vi "VI server_Set Controls Property from String Format_Array Input.vi"(4 "Property":T1="Value", 7 "Labels":string[](array[string]), 8 "error in (no error)":errorcluster, 9 "Values":string[](array[string]), 11 "VI Server.RefsCluster":T2 caption="VI Server Cluster") -> (0 "error out":errorcluster, 3 "VI Server Cluster.DUP":T2)   [LabVIEW 2020]
doc: "Sets specified property of the multiple controls (labels array input) to values formatted as strings."
uses:
  VI Server_TypeDefs/VI Server_RefsCluster.ctl
  VI Server Libraries/VI Server Controls.llb/VI Server_Properties.ctl
  VI Server Toolkit LV2013.lvlib
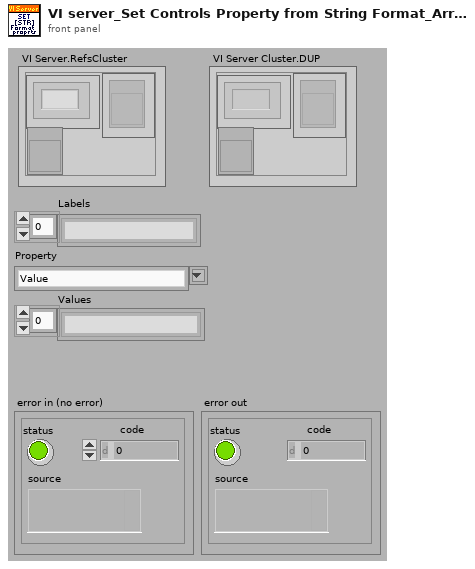
[diagram p1: front panel]
types:
  T1 = typedef "VI Server Toolkit LV2013.lvlib/VI Server_Properties.ctl" = string
  T2 = typedef "VI Server_RefsCluster.ctl" = cluster{"Labels":string[], "Refs":refnum<vi>[], "VI Ref":refnum<vi>}
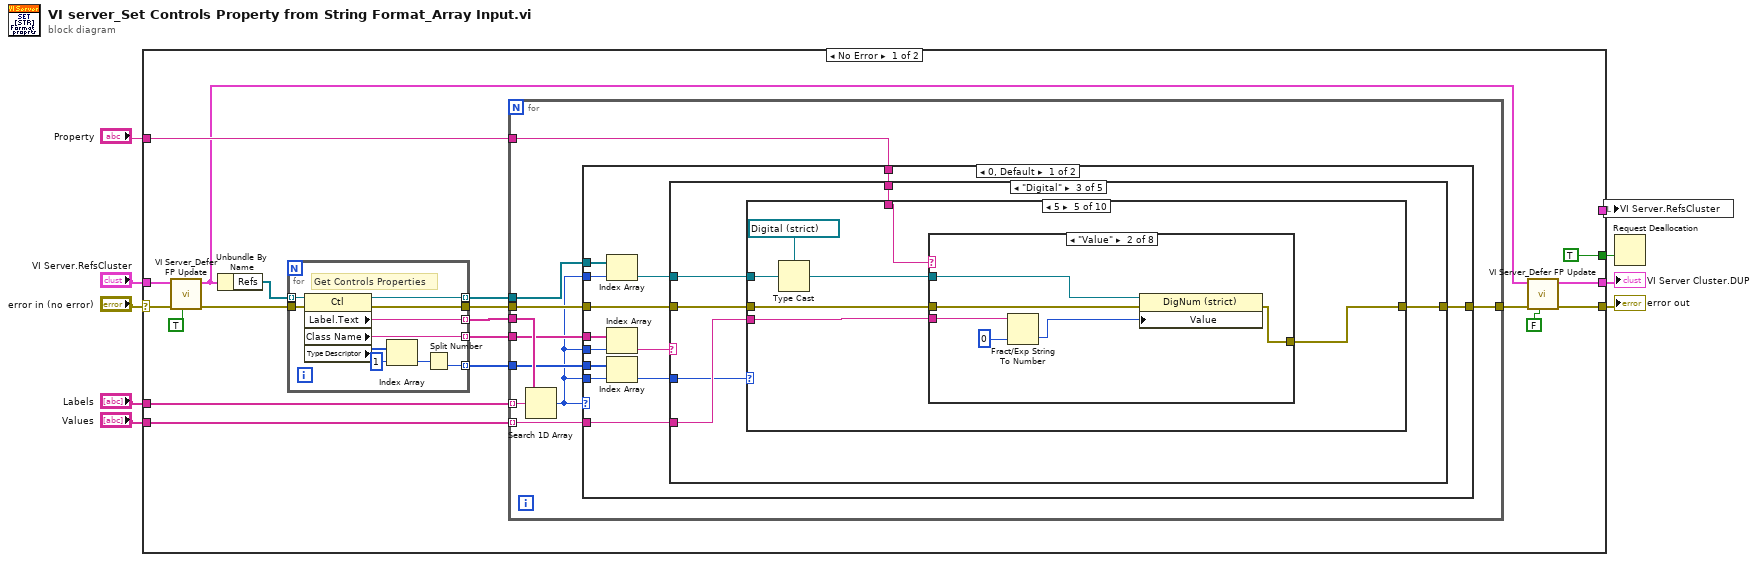
[diagram p0: block diagram]
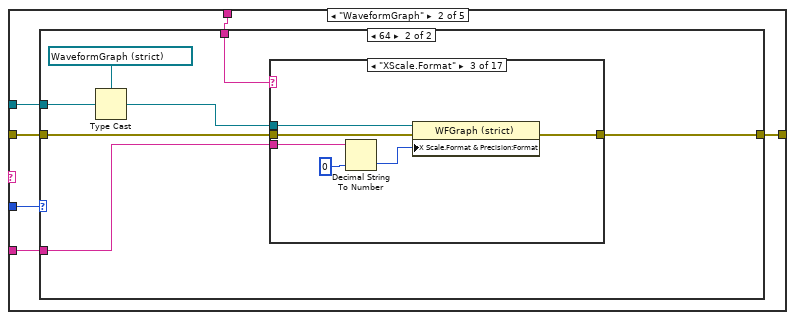
[diagram p3: hidden frame]
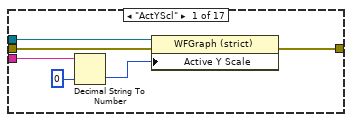
[diagram p5: hidden frame]
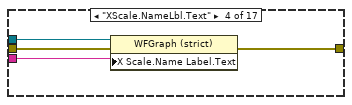
[diagram p7: hidden frame]
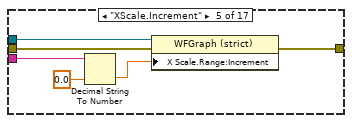
[diagram p8: hidden frame]
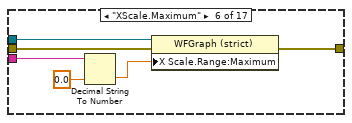
[diagram p9: hidden frame]
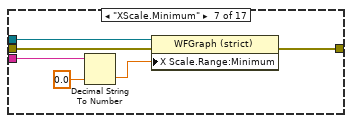
[diagram p10: hidden frame]
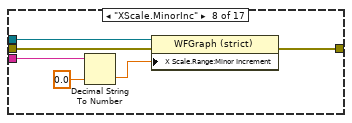
[diagram p11: hidden frame]
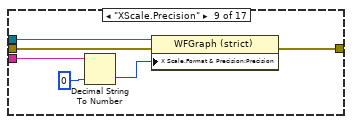
[diagram p12: hidden frame]
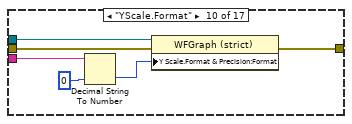
[diagram p13: hidden frame]
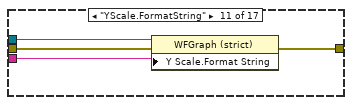
[diagram p14: hidden frame]
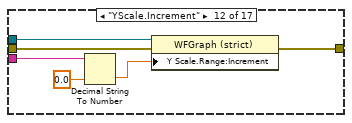
[diagram p15: hidden frame]
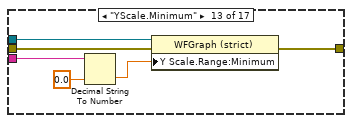
[diagram p16: hidden frame]
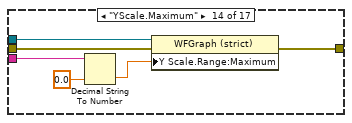
[diagram p17: hidden frame]
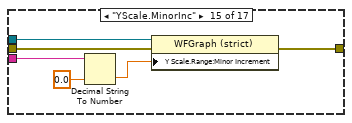
[diagram p18: hidden frame]
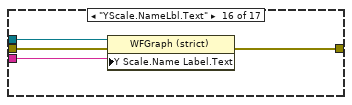
[diagram p19: hidden frame]
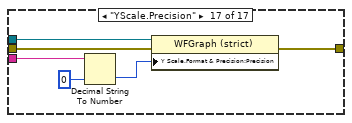
[diagram p20: hidden frame]
diagram:
  n1 = case shown="No Error" "error in (no error)" {
    selector: "error in (no error)" -> [w20 w1359]
    tunnel: "Labels" -> [w22 _]
    tunnel: "Values" -> [w23 _]
    tunnel: [w16 w1359] -> w7
    tunnel: "VI Server.RefsCluster" -> [w18 _]
    tunnel: "Property" -> [w13 _]
    tunnel: [w12 _] -> w3
    tunnel: [TRUE _] -> w2
    tunnel: [_ w1358] -> w1
    frame No Error {
      n2 = call "VI Server_Defer FP Update.vi"("Defer Panel Updates? (F)"=TRUE ("Defer Panel Updates (F)"), "error in"=w20, "VI Server Cluster"=w18) -> ("error out"=w19:errorcluster, "VI Server Cluster.DUP"=w10:T2)  [unwired: 7 out]
      n3 = Unbundle By Name(w10) -> ("Refs"=w21:refnum<vi>[])
      n4 = for {
        tunnel: w21 -> [w1357] mode=indexing
        tunnel: w19 -> [w1356]
        tunnel: [w1355] -> w28 mode=indexing
        tunnel: [w1354] -> w26 mode=indexing
        tunnel: [w1353] -> w27 mode=indexing
        tunnel: [w1352] -> w25
        tunnel: [w1348] -> w24 mode=indexing
        # "Get Controls Properties"
        n5 = property class="Ctl"(reference=w1357, error in=w1356) -> (reference out=w1353:refnum<vi>, error out=w1352:errorcluster, "Label.Text"=w1355:string, "Class Name"=w1354:string, "Type Descriptor"=w1351:i16[])
        n6 = Index Array(array=w1351, index=1) -> (element=w1349:i16)
        n7 = Split Number(x=w1349) -> (lo(x)=w1348:u8)  [unwired: 1 out]
      }
      n8 = for {
        tunnel: w22 -> [w36] mode=indexing
        tunnel: w28 -> [w38]
        tunnel: w27 -> [w34]
        tunnel: w26 -> [w37]
        tunnel: w23 -> [w35] mode=indexing
        tunnel: w25 -> [w33]
        tunnel: [w32] -> w15
        tunnel: w24 -> [w31]
        tunnel: w13 -> [w29]
        n9 = Search 1D Array(1D array=w38, element=w36) -> (index of element=w30:i32)  [unwired: 1 out]
        n10 = case shown="0, Default" w30 {
          tunnel: w34 -> [w51 _]
          tunnel: w30 -> [w50 _]
          tunnel: w37 -> [w49 _]
          tunnel: w30 -> [w48 _]
          tunnel: w35 -> [w45 _]
          tunnel: w33 -> [w44 w1347]
          tunnel: [w43 w1347] -> w32
          tunnel: w31 -> [w42 _]
          tunnel: w30 -> [w41 _]
          tunnel: w29 -> [w39 _]
          frame 0, Default {
            n11 = Index Array(array=w51, index=w50) -> (element=w46:refnum<vi>)
            n12 = Index Array(array=w49, index=w48) -> (element=w47:string)
            n13 = Index Array(array=w42, index=w41) -> (element=w40:u8)
            n14 = case shown="\"Digital\"" w47 {
              tunnel: w46 -> [_ w56 w161 w623 w1333]
              tunnel: w45 -> [_ w54 w160 w622 w1331]
              tunnel: w44 -> [w52 w57 w163 w625 w1335]
              tunnel: [w52 w53 w162 w624 w1334] -> w43
              tunnel: w40 -> [_ w58 w159 w621 _]
              tunnel: w39 -> [_ w55 w158 w620 w1329]
              frame "", Default {
              }
              frame "WaveformGraph" {
                n15 = case shown="64" w58 {
                  tunnel: w57 -> [w59 w63]
                  tunnel: w56 -> [_ w66]
                  tunnel: w55 -> [_ w62]
                  tunnel: w54 -> [_ w61]
                  tunnel: [w59 w60] -> w53
                  frame 0, Default {
                  }
                  frame 64 {
                    n16 = Type Cast(type=refnum<vi> refnum ("XY Graph"), x=w66) -> (*(type *) &x=w64:refnum<vi>)
                    n17 = case shown="\"XScale.Format\"" w62 {
                      tunnel: w64 -> [w72 _ w79 w83 w89 w95 w101 w107 w113 w119 w123 w129 w135 w141 w147 w151 w157]
                      tunnel: w63 -> [w71 w73 w78 w82 w88 w94 w100 w106 w112 w118 w122 w128 w134 w140 w146 w150 w156]
                      tunnel: w61 -> [w70 _ w76 w80 w86 w92 w98 w104 w110 w116 w120 w126 w132 w138 w144 w148 w154]
                      tunnel: [w69 w73 w77 w81 w87 w93 w99 w105 w111 w117 w121 w127 w133 w139 w145 w149 w155] -> w60
                      frame "ActYScl" {
                        n18 = Decimal String To Number(string=w70, default (0L)=0 ("Active Y Scale")) -> (number=w67:i32)  [unwired: 2 out]
                        n19 = property class="WFGraph (strict)"(reference=w72, error in=w71, "Active Y Scale"=w67) -> (error out=w69:errorcluster)  [unwired: 1 out]
                      }
                      frame "False", Default {
                      }
                      frame "XScale.Format" {
                        n20 = Decimal String To Number(string=w76, default (0L)=u8 0 ("Y Scale.Format & Precision:Format")) -> (number=w75:u8)  [unwired: 2 out]
                        n21 = property class="WFGraph (strict)"(reference=w79, error in=w78, "X Scale.Format & Precision:Format"=w75) -> (error out=w77:errorcluster)  [unwired: 1 out]
                      }
                      frame "XScale.NameLbl.Text" {
                        n22 = property class="WFGraph (strict)"(reference=w83, error in=w82, "X Scale.Name Label.Text"=w80) -> (error out=w81:errorcluster)  [unwired: 1 out]
                      }
                      frame "XScale.Increment" {
                        n23 = Decimal String To Number(string=w86, default (0L)=0.0 ("X Scale.Range:Minimum")) -> (number=w84:dbl)  [unwired: 2 out]
                        n24 = property class="WFGraph (strict)"(reference=w89, error in=w88, "X Scale.Range:Increment"=w84) -> (error out=w87:errorcluster)  [unwired: 1 out]
                      }
                      frame "XScale.Maximum" {
                        n25 = Decimal String To Number(string=w92, default (0L)=0.0 ("X Scale.Range:Minimum")) -> (number=w90:dbl)  [unwired: 2 out]
                        n26 = property class="WFGraph (strict)"(reference=w95, error in=w94, "X Scale.Range:Maximum"=w90) -> (error out=w93:errorcluster)  [unwired: 1 out]
                      }
                      frame "XScale.Minimum" {
                        n27 = Decimal String To Number(string=w98, default (0L)=0.0 ("X Scale.Range:Minimum")) -> (number=w96:dbl)  [unwired: 2 out]
                        n28 = property class="WFGraph (strict)"(reference=w101, error in=w100, "X Scale.Range:Minimum"=w96) -> (error out=w99:errorcluster)  [unwired: 1 out]
                      }
                      frame "XScale.MinorInc" {
                        n29 = Decimal String To Number(string=w104, default (0L)=0.0 ("X Scale.Range:Minimum")) -> (number=w102:dbl)  [unwired: 2 out]
                        n30 = property class="WFGraph (strict)"(reference=w107, error in=w106, "X Scale.Range:Minor Increment"=w102) -> (error out=w105:errorcluster)  [unwired: 1 out]
                      }
                      frame "XScale.Precision" {
                        n31 = Decimal String To Number(string=w110, default (0L)=u8 0 ("Y Scale.Format & Precision:Format")) -> (number=w109:u8)  [unwired: 2 out]
                        n32 = property class="WFGraph (strict)"(reference=w113, error in=w112, "X Scale.Format & Precision:Precision"=w109) -> (error out=w111:errorcluster)  [unwired: 1 out]
                      }
                      frame "YScale.Format" {
                        n33 = Decimal String To Number(string=w116, default (0L)=u8 0 ("Y Scale.Format & Precision:Format")) -> (number=w115:u8)  [unwired: 2 out]
                        n34 = property class="WFGraph (strict)"(reference=w119, error in=w118, "Y Scale.Format & Precision:Format"=w115) -> (error out=w117:errorcluster)  [unwired: 1 out]
                      }
                      frame "YScale.FormatString" {
                        n35 = property class="WFGraph (strict)"(reference=w123, error in=w122, "Y Scale.Format String"=w120) -> (error out=w121:errorcluster)  [unwired: 1 out]
                      }
                      frame "YScale.Increment" {
                        n36 = Decimal String To Number(string=w126, default (0L)=0.0 ("X Scale.Range:Minimum")) -> (number=w124:dbl)  [unwired: 2 out]
                        n37 = property class="WFGraph (strict)"(reference=w129, error in=w128, "Y Scale.Range:Increment"=w124) -> (error out=w127:errorcluster)  [unwired: 1 out]
                      }
                      frame "YScale.Minimum" {
                        n38 = Decimal String To Number(string=w132, default (0L)=0.0 ("X Scale.Range:Minimum")) -> (number=w130:dbl)  [unwired: 2 out]
                        n39 = property class="WFGraph (strict)"(reference=w135, error in=w134, "Y Scale.Range:Minimum"=w130) -> (error out=w133:errorcluster)  [unwired: 1 out]
                      }
                      frame "YScale.Maximum" {
                        n40 = Decimal String To Number(string=w138, default (0L)=0.0 ("X Scale.Range:Minimum")) -> (number=w136:dbl)  [unwired: 2 out]
                        n41 = property class="WFGraph (strict)"(reference=w141, error in=w140, "Y Scale.Range:Maximum"=w136) -> (error out=w139:errorcluster)  [unwired: 1 out]
                      }
                      frame "YScale.MinorInc" {
                        n42 = Decimal String To Number(string=w144, default (0L)=0.0 ("X Scale.Range:Minimum")) -> (number=w142:dbl)  [unwired: 2 out]
                        n43 = property class="WFGraph (strict)"(reference=w147, error in=w146, "Y Scale.Range:Minor Increment"=w142) -> (error out=w145:errorcluster)  [unwired: 1 out]
                      }
                      frame "YScale.NameLbl.Text" {
                        n44 = property class="WFGraph (strict)"(reference=w151, error in=w150, "Y Scale.Name Label.Text"=w148) -> (error out=w149:errorcluster)  [unwired: 1 out]
                      }
                      frame "YScale.Precision" {
                        n45 = Decimal String To Number(string=w154, default (0L)=u8 0 ("Y Scale.Format & Precision:Format")) -> (number=w153:u8)  [unwired: 2 out]
                        n46 = property class="WFGraph (strict)"(reference=w157, error in=w156, "Y Scale.Format & Precision:Precision"=w153) -> (error out=w155:errorcluster)  [unwired: 1 out]
                      }
                    }
                  }
                }
              }
              frame "Digital" {
                n47 = case shown="5" w159 {
                  tunnel: w163 -> [w164 w171 w216 w260 w312 w359 w412 w460 w510 w570]
                  tunnel: [w164 w170 w212 w262 w315 w361 w410 w458 w512 w569] -> w162
                  tunnel: w161 -> [_ w169 w218 w266 w317 w365 w416 w464 w516 w574]
                  tunnel: w160 -> [_ w167 w215 w261 w311 w360 w411 w459 w511 w568]
                  tunnel: w158 -> [_ w165 w214 w264 w314 w363 w414 w461 w514 w572]
                  frame 0, Default {
                  }
                  frame 1 {
                    n48 = Type Cast(type=refnum<vi> refnum ("I8"), x=w169) -> (*(type *) &x=w168:refnum<vi>)
                    n49 = case shown="\"Format\"" w165 {
                      tunnel: w171 -> [w172 w178 w185 w192 w198 w205 w211]
                      tunnel: [w172 w177 w184 w191 w197 w204 w210] -> w170
                      tunnel: w168 -> [_ w176 w183 w190 w196 w203 w209]
                      tunnel: w167 -> [_ w175 w182 w189 w195 w202 w208]
                      frame "False", Default {
                      }
                      frame "Minimum" {
                        n50 = Fract/Exp String To Number(string=w175, default (0 dbl)=0.0 ("Data Range:Minimum")) -> (number=w173:dbl)  [unwired: 3 out]
                        n51 = property class="DigNum (strict)"(reference=w176, error in=w178, "Data Range:Minimum"=w173) -> (reference out=w179:refnum<vi>, error out=w177:errorcluster)
                        n52 = Close Reference(reference=w179) -> ()  [unwired: 1 in, 1 out]
                      }
                      frame "Maximum" {
                        n53 = Fract/Exp String To Number(string=w182, default (0 dbl)=0.0 ("Data Range:Minimum")) -> (number=w180:dbl)  [unwired: 3 out]
                        n54 = property class="DigNum (strict)"(reference=w183, error in=w185, "Data Range:Maximum"=w180) -> (reference out=w186:refnum<vi>, error out=w184:errorcluster)
                        n55 = Close Reference(reference=w186) -> ()  [unwired: 1 in, 1 out]
                      }
                      frame "Increment" {
                        n56 = Fract/Exp String To Number(string=w189, default (0 dbl)=0.0 ("Data Range:Minimum")) -> (number=w187:dbl)  [unwired: 3 out]
                        n57 = property class="DigNum (strict)"(reference=w190, error in=w192, "Data Range:Increment"=w187) -> (reference out=w193:refnum<vi>, error out=w191:errorcluster)
                        n58 = Close Reference(reference=w193) -> ()  [unwired: 1 in, 1 out]
                      }
                      frame "Format String" {
                        n59 = property class="DigNum (strict)"(reference=w196, error in=w198, "Format String"=w195) -> (reference out=w194:refnum<vi>, error out=w197:errorcluster)
                        n60 = Close Reference(reference=w194) -> ()  [unwired: 1 in, 1 out]
                      }
                      frame "Format" {
                        n61 = Decimal String To Number(string=w202, default (0L)=u8 0 ("Format & Precision:Format")) -> (number=w200:u8)  [unwired: 2 out]
                        n62 = property class="DigNum (strict)"(reference=w203, error in=w205, "Format & Precision:Format"=w200) -> (reference out=w199:refnum<vi>, error out=w204:errorcluster)
                        n63 = Close Reference(reference=w199) -> ()  [unwired: 1 in, 1 out]
                      }
                      frame "Precision" {
                        n64 = Decimal String To Number(string=w208, default (0L)=u8 0 ("Format & Precision:Format")) -> (number=w206:u8)  [unwired: 2 out]
                        n65 = property class="DigNum (strict)"(reference=w209, error in=w211, "Format & Precision:Precision"=w206) -> (error out=w210:errorcluster)  [unwired: 1 out]
                      }
                    }
                  }
                  frame 2 {
                    n66 = Type Cast(type=refnum<vi> refnum ("I16"), x=w218) -> (*(type *) &x=w213:refnum<vi>)
                    n67 = case shown="\"Format\"" w214 {
                      tunnel: w216 -> [w219 w225 w231 w237 w243 w247 w253 w259]
                      tunnel: [w219 w224 w230 w236 w242 w246 w252 w258] -> w212
                      tunnel: w213 -> [_ w223 w229 w235 w241 w245 w251 w257]
                      tunnel: w215 -> [_ w222 w228 w234 w240 w244 w250 w256]
                      frame "False", Default {
                      }
                      frame "Value" {
                        n68 = Fract/Exp String To Number(string=w222, default (0 dbl)=i16 0) -> (number=w221:i16)  [unwired: 3 out]
                        n69 = property class="DigNum (strict)"(reference=w223, error in=w225, "Value"=w221) -> (error out=w224:errorcluster)  [unwired: 1 out]
                      }
                      frame "Minimum" {
                        n70 = Fract/Exp String To Number(string=w228, default (0 dbl)=0.0 ("Data Range:Minimum")) -> (number=w226:dbl)  [unwired: 3 out]
                        n71 = property class="DigNum (strict)"(reference=w229, error in=w231, "Data Range:Minimum"=w226) -> (error out=w230:errorcluster)  [unwired: 1 out]
                      }
                      frame "Maximum" {
                        n72 = Fract/Exp String To Number(string=w234, default (0 dbl)=0.0 ("Data Range:Minimum")) -> (number=w232:dbl)  [unwired: 3 out]
                        n73 = property class="DigNum (strict)"(reference=w235, error in=w237, "Data Range:Maximum"=w232) -> (error out=w236:errorcluster)  [unwired: 1 out]
                      }
                      frame "Increment" {
                        n74 = Fract/Exp String To Number(string=w240, default (0 dbl)=0.0 ("Data Range:Minimum")) -> (number=w238:dbl)  [unwired: 3 out]
                        n75 = property class="DigNum (strict)"(reference=w241, error in=w243, "Data Range:Increment"=w238) -> (error out=w242:errorcluster)  [unwired: 1 out]
                      }
                      frame "Format String" {
                        n76 = property class="DigNum (strict)"(reference=w245, error in=w247, "Format String"=w244) -> (error out=w246:errorcluster)  [unwired: 1 out]
                      }
                      frame "Format" {
                        n77 = Decimal String To Number(string=w250, default (0L)=u8 0 ("Format & Precision:Format")) -> (number=w248:u8)  [unwired: 2 out]
                        n78 = property class="DigNum (strict)"(reference=w251, error in=w253, "Format & Precision:Format"=w248) -> (error out=w252:errorcluster)  [unwired: 1 out]
                      }
                      frame "Precision" {
                        n79 = Decimal String To Number(string=w256, default (0L)=u8 0 ("Format & Precision:Format")) -> (number=w254:u8)  [unwired: 2 out]
                        n80 = property class="DigNum (strict)"(reference=w257, error in=w259, "Format & Precision:Precision"=w254) -> (error out=w258:errorcluster)  [unwired: 1 out]
                      }
                    }
                  }
                  frame 3 {
                    n81 = Type Cast(type=refnum<vi> refnum ("I32"), x=w266) -> (*(type *) &x=w263:refnum<vi>)
                    n82 = case shown="\"Value\"" w264 {
                      tunnel: w260 -> [w267 w273 w279 w286 w293 w298 w304 w310]
                      tunnel: [w267 w272 w278 w285 w292 w297 w303 w309] -> w262
                      tunnel: w263 -> [_ w271 w277 w284 w291 w296 w302 w308]
                      tunnel: w261 -> [_ w270 w276 w283 w290 w295 w301 w307]
                      frame "False", Default {
                      }
                      frame "Value" {
                        n83 = Fract/Exp String To Number(string=w270, default (0 dbl)=0) -> (number=w269:i32)  [unwired: 3 out]
                        n84 = property class="DigNum (strict)"(reference=w271, error in=w273, "Value"=w269) -> (error out=w272:errorcluster)  [unwired: 1 out]
                      }
                      frame "Minimum" {
                        n85 = Fract/Exp String To Number(string=w276, default (0 dbl)=0.0 ("Data Range:Minimum")) -> (number=w274:dbl)  [unwired: 3 out]
                        n86 = property class="DigNum (strict)"(reference=w277, error in=w279, "Data Range:Minimum"=w274) -> (reference out=w280:refnum<vi>, error out=w278:errorcluster)
                        n87 = Close Reference(reference=w280) -> ()  [unwired: 1 in, 1 out]
                      }
                      frame "Maximum" {
                        n88 = Fract/Exp String To Number(string=w283, default (0 dbl)=0.0 ("Data Range:Minimum")) -> (number=w281:dbl)  [unwired: 3 out]
                        n89 = property class="DigNum (strict)"(reference=w284, error in=w286, "Data Range:Maximum"=w281) -> (reference out=w287:refnum<vi>, error out=w285:errorcluster)
                        n90 = Close Reference(reference=w287) -> ()  [unwired: 1 in, 1 out]
                      }
                      frame "Increment" {
                        n91 = Fract/Exp String To Number(string=w290, default (0 dbl)=0.0 ("Data Range:Minimum")) -> (number=w288:dbl)  [unwired: 3 out]
                        n92 = property class="DigNum (strict)"(reference=w291, error in=w293, "Data Range:Increment"=w288) -> (reference out=w294:refnum<vi>, error out=w292:errorcluster)
                        n93 = Close Reference(reference=w294) -> ()  [unwired: 1 in, 1 out]
                      }
                      frame "Format String" {
                        n94 = property class="DigNum (strict)"(reference=w296, error in=w298, "Format String"=w295) -> (error out=w297:errorcluster)  [unwired: 1 out]
                      }
                      frame "Format" {
                        n95 = Decimal String To Number(string=w301, default (0L)=u8 0 ("Format & Precision:Format")) -> (number=w299:u8)  [unwired: 2 out]
                        n96 = property class="DigNum (strict)"(reference=w302, error in=w304, "Format & Precision:Format"=w299) -> (error out=w303:errorcluster)  [unwired: 1 out]
                      }
                      frame "Precision" {
                        n97 = Decimal String To Number(string=w307, default (0L)=u8 0 ("Format & Precision:Format")) -> (number=w305:u8)  [unwired: 2 out]
                        n98 = property class="DigNum (strict)"(reference=w308, error in=w310, "Format & Precision:Precision"=w305) -> (error out=w309:errorcluster)  [unwired: 1 out]
                      }
                    }
                  }
                  frame 5 {
                    n99 = Type Cast(type=refnum<vi> refnum ("U8"), x=w317) -> (*(type *) &x=w313:refnum<vi>)
                    n100 = case shown="\"Value\"" w314 {
                      tunnel: w312 -> [w318 w324 w330 w336 w342 w346 w352 w358]
                      tunnel: [w318 w323 w329 w335 w341 w345 w351 w357] -> w315
                      tunnel: w313 -> [_ w322 w328 w334 w340 w344 w350 w356]
                      tunnel: w311 -> [_ w321 w327 w333 w339 w343 w349 w355]
                      frame "False", Default {
                      }
                      frame "Value" {
                        n101 = Fract/Exp String To Number(string=w321, default (0 dbl)=u8 0) -> (number=w320:u8)  [unwired: 3 out]
                        n102 = property class="DigNum (strict)"(reference=w322, error in=w324, "Value"=w320) -> (error out=w323:errorcluster)  [unwired: 1 out]
                      }
                      frame "Minimum" {
                        n103 = Fract/Exp String To Number(string=w327, default (0 dbl)=0.0 ("Data Range:Minimum")) -> (number=w325:dbl)  [unwired: 3 out]
                        n104 = property class="DigNum (strict)"(reference=w328, error in=w330, "Data Range:Minimum"=w325) -> (error out=w329:errorcluster)  [unwired: 1 out]
                      }
                      frame "Maximum" {
                        n105 = Fract/Exp String To Number(string=w333, default (0 dbl)=0.0 ("Data Range:Minimum")) -> (number=w331:dbl)  [unwired: 3 out]
                        n106 = property class="DigNum (strict)"(reference=w334, error in=w336, "Data Range:Maximum"=w331) -> (error out=w335:errorcluster)  [unwired: 1 out]
                      }
                      frame "Increment" {
                        n107 = Fract/Exp String To Number(string=w339, default (0 dbl)=0.0 ("Data Range:Minimum")) -> (number=w337:dbl)  [unwired: 3 out]
                        n108 = property class="DigNum (strict)"(reference=w340, error in=w342, "Data Range:Increment"=w337) -> (error out=w341:errorcluster)  [unwired: 1 out]
                      }
                      frame "Format String" {
                        n109 = property class="DigNum (strict)"(reference=w344, error in=w346, "Format String"=w343) -> (error out=w345:errorcluster)  [unwired: 1 out]
                      }
                      frame "Format" {
                        n110 = Decimal String To Number(string=w349, default (0L)=u8 0 ("Format & Precision:Format")) -> (number=w347:u8)  [unwired: 2 out]
                        n111 = property class="DigNum (strict)"(reference=w350, error in=w352, "Format & Precision:Format"=w347) -> (error out=w351:errorcluster)  [unwired: 1 out]
                      }
                      frame "Precision" {
                        n112 = Decimal String To Number(string=w355, default (0L)=u8 0 ("Format & Precision:Format")) -> (number=w353:u8)  [unwired: 2 out]
                        n113 = property class="DigNum (strict)"(reference=w356, error in=w358, "Format & Precision:Precision"=w353) -> (error out=w357:errorcluster)  [unwired: 1 out]
                      }
                    }
                  }
                  frame 6 {
                    n114 = Type Cast(type=refnum<vi> refnum ("U16"), x=w365) -> (*(type *) &x=w362:refnum<vi>)
                    n115 = case shown="\"Value\"" w363 {
                      tunnel: w359 -> [w366 w372 w378 w385 w392 w397 w403 w409]
                      tunnel: [w366 w371 w377 w384 w391 w396 w402 w408] -> w361
                      tunnel: w362 -> [_ w370 w376 w383 w390 w395 w401 w407]
                      tunnel: w360 -> [_ w369 w375 w382 w389 w394 w400 w406]
                      frame "False", Default {
                      }
                      frame "Value" {
                        n116 = Fract/Exp String To Number(string=w369, default (0 dbl)=u16 0) -> (number=w368:u16)  [unwired: 3 out]
                        n117 = property class="DigNum (strict)"(reference=w370, error in=w372, "Value"=w368) -> (error out=w371:errorcluster)  [unwired: 1 out]
                      }
                      frame "Minimum" {
                        n118 = Fract/Exp String To Number(string=w375, default (0 dbl)=0.0 ("Data Range:Minimum")) -> (number=w373:dbl)  [unwired: 3 out]
                        n119 = property class="DigNum (strict)"(reference=w376, error in=w378, "Data Range:Minimum"=w373) -> (reference out=w379:refnum<vi>, error out=w377:errorcluster)
                        n120 = Close Reference(reference=w379) -> ()  [unwired: 1 in, 1 out]
                      }
                      frame "Maximum" {
                        n121 = Fract/Exp String To Number(string=w382, default (0 dbl)=0.0 ("Data Range:Minimum")) -> (number=w380:dbl)  [unwired: 3 out]
                        n122 = property class="DigNum (strict)"(reference=w383, error in=w385, "Data Range:Maximum"=w380) -> (reference out=w386:refnum<vi>, error out=w384:errorcluster)
                        n123 = Close Reference(reference=w386) -> ()  [unwired: 1 in, 1 out]
                      }
                      frame "Increment" {
                        n124 = Fract/Exp String To Number(string=w389, default (0 dbl)=0.0 ("Data Range:Minimum")) -> (number=w387:dbl)  [unwired: 3 out]
                        n125 = property class="DigNum (strict)"(reference=w390, error in=w392, "Data Range:Increment"=w387) -> (reference out=w393:refnum<vi>, error out=w391:errorcluster)
                        n126 = Close Reference(reference=w393) -> ()  [unwired: 1 in, 1 out]
                      }
                      frame "Format String" {
                        n127 = property class="DigNum (strict)"(reference=w395, error in=w397, "Format String"=w394) -> (error out=w396:errorcluster)  [unwired: 1 out]
                      }
                      frame "Format" {
                        n128 = Decimal String To Number(string=w400, default (0L)=u8 0 ("Format & Precision:Format")) -> (number=w398:u8)  [unwired: 2 out]
                        n129 = property class="DigNum (strict)"(reference=w401, error in=w403, "Format & Precision:Format"=w398) -> (error out=w402:errorcluster)  [unwired: 1 out]
                      }
                      frame "Precision" {
                        n130 = Decimal String To Number(string=w406, default (0L)=u8 0 ("Format & Precision:Format")) -> (number=w404:u8)  [unwired: 2 out]
                        n131 = property class="DigNum (strict)"(reference=w407, error in=w409, "Format & Precision:Precision"=w404) -> (error out=w408:errorcluster)  [unwired: 1 out]
                      }
                    }
                  }
                  frame 7 {
                    n132 = Type Cast(type=refnum<vi> refnum ("U32"), x=w416) -> (*(type *) &x=w413:refnum<vi>)
                    n133 = case shown="\"Value\"" w414 {
                      tunnel: w412 -> [w417 w423 w429 w435 w441 w445 w451 w457]
                      tunnel: [w417 w422 w428 w434 w440 w444 w450 w456] -> w410
                      tunnel: w413 -> [_ w421 w427 w433 w439 w443 w449 w455]
                      tunnel: w411 -> [_ w420 w426 w432 w438 w442 w448 w454]
                      frame "False", Default {
                      }
                      frame "Value" {
                        n134 = Fract/Exp String To Number(string=w420, default (0 dbl)=u32 0) -> (number=w419:u32)  [unwired: 3 out]
                        n135 = property class="DigNum (strict)"(reference=w421, error in=w423, "Value"=w419) -> (error out=w422:errorcluster)  [unwired: 1 out]
                      }
                      frame "Minimum" {
                        n136 = Fract/Exp String To Number(string=w426, default (0 dbl)=0.0 ("Data Range:Minimum")) -> (number=w424:dbl)  [unwired: 3 out]
                        n137 = property class="DigNum (strict)"(reference=w427, error in=w429, "Data Range:Minimum"=w424) -> (error out=w428:errorcluster)  [unwired: 1 out]
                      }
                      frame "Maximum" {
                        n138 = Fract/Exp String To Number(string=w432, default (0 dbl)=0.0 ("Data Range:Minimum")) -> (number=w430:dbl)  [unwired: 3 out]
                        n139 = property class="DigNum (strict)"(reference=w433, error in=w435, "Data Range:Maximum"=w430) -> (error out=w434:errorcluster)  [unwired: 1 out]
                      }
                      frame "Increment" {
                        n140 = Fract/Exp String To Number(string=w438, default (0 dbl)=0.0 ("Data Range:Minimum")) -> (number=w436:dbl)  [unwired: 3 out]
                        n141 = property class="DigNum (strict)"(reference=w439, error in=w441, "Data Range:Increment"=w436) -> (error out=w440:errorcluster)  [unwired: 1 out]
                      }
                      frame "Format String" {
                        n142 = property class="DigNum (strict)"(reference=w443, error in=w445, "Format String"=w442) -> (error out=w444:errorcluster)  [unwired: 1 out]
                      }
                      frame "Format" {
                        n143 = Decimal String To Number(string=w448, default (0L)=u8 0 ("Format & Precision:Format")) -> (number=w446:u8)  [unwired: 2 out]
                        n144 = property class="DigNum (strict)"(reference=w449, error in=w451, "Format & Precision:Format"=w446) -> (error out=w450:errorcluster)  [unwired: 1 out]
                      }
                      frame "Precision" {
                        n145 = Decimal String To Number(string=w454, default (0L)=u8 0 ("Format & Precision:Format")) -> (number=w452:u8)  [unwired: 2 out]
                        n146 = property class="DigNum (strict)"(reference=w455, error in=w457, "Format & Precision:Precision"=w452) -> (error out=w456:errorcluster)  [unwired: 1 out]
                      }
                    }
                  }
                  frame 9 {
                    n147 = Type Cast(type=refnum<vi> refnum ("SGL"), x=w464) -> (*(type *) &x=w462:refnum<vi>)
                    n148 = case shown="\"Value\"" w461 {
                      tunnel: w460 -> [w465 w475 w481 w487 w493 w497 w503 w509]
                      tunnel: [w465 w474 w480 w486 w492 w496 w502 w508] -> w458
                      tunnel: w462 -> [_ w473 w479 w485 w491 w495 w501 w507]
                      tunnel: w459 -> [_ w468 w478 w484 w490 w494 w500 w506]
                      frame "False", Default {
                      }
                      frame "Value" {
                        n149 = Empty String/Path?(string/path=w468) -> (empty?=w471:bool)
                        n150 = Not(x=w471) -> (.not. x?=w470:bool)
                        n151 = Fract/Exp String To Number(string=w468, default (0 dbl)=sgl 0.0) -> (number=w467:sgl)  [unwired: 3 out]
                        n152 = Select(t=w467, s=w470, f=sgl nan) -> (s? t:f=w466:sgl)
                        n153 = property class="DigNum (strict)"(reference=w473, error in=w475, "Value"=w466) -> (error out=w474:errorcluster)  [unwired: 1 out]
                      }
                      frame "Minimum" {
                        n154 = Fract/Exp String To Number(string=w478, default (0 dbl)=0.0 ("Data Range:Minimum")) -> (number=w476:dbl)  [unwired: 3 out]
                        n155 = property class="DigNum (strict)"(reference=w479, error in=w481, "Data Range:Minimum"=w476) -> (error out=w480:errorcluster)  [unwired: 1 out]
                      }
                      frame "Maximum" {
                        n156 = Fract/Exp String To Number(string=w484, default (0 dbl)=0.0 ("Data Range:Minimum")) -> (number=w482:dbl)  [unwired: 3 out]
                        n157 = property class="DigNum (strict)"(reference=w485, error in=w487, "Data Range:Maximum"=w482) -> (error out=w486:errorcluster)  [unwired: 1 out]
                      }
                      frame "Increment" {
                        n158 = Fract/Exp String To Number(string=w490, default (0 dbl)=0.0 ("Data Range:Minimum")) -> (number=w488:dbl)  [unwired: 3 out]
                        n159 = property class="DigNum (strict)"(reference=w491, error in=w493, "Data Range:Increment"=w488) -> (error out=w492:errorcluster)  [unwired: 1 out]
                      }
                      frame "Format String" {
                        n160 = property class="DigNum (strict)"(reference=w495, error in=w497, "Format String"=w494) -> (error out=w496:errorcluster)  [unwired: 1 out]
                      }
                      frame "Format" {
                        n161 = Decimal String To Number(string=w500, default (0L)=u8 0 ("Format & Precision:Format")) -> (number=w498:u8)  [unwired: 2 out]
                        n162 = property class="DigNum (strict)"(reference=w501, error in=w503, "Format & Precision:Format"=w498) -> (error out=w502:errorcluster)  [unwired: 1 out]
                      }
                      frame "Precision" {
                        n163 = Decimal String To Number(string=w506, default (0L)=u8 0 ("Format & Precision:Format")) -> (number=w504:u8)  [unwired: 2 out]
                        n164 = property class="DigNum (strict)"(reference=w507, error in=w509, "Format & Precision:Precision"=w504) -> (error out=w508:errorcluster)  [unwired: 1 out]
                      }
                    }
                  }
                  frame 10 {
                    n165 = Type Cast(type=refnum<vi> refnum ("DBL"), x=w516) -> (*(type *) &x=w513:refnum<vi>)
                    n166 = case shown="\"Value\"" w514 {
                      tunnel: w510 -> [w517 w523 w528 w535 w542 w549 w556 w567]
                      tunnel: [w517 w522 w527 w534 w541 w548 w555 w566] -> w512
                      tunnel: w513 -> [_ w521 w526 w533 w540 w547 w554 w565]
                      tunnel: w511 -> [_ w520 w525 w532 w539 w546 w553 w563]
                      frame "False", Default {
                      }
                      frame "Format" {
                        n167 = Decimal String To Number(string=w520, default (0L)=u8 0 ("Format & Precision:Format")) -> (number=w518:u8)  [unwired: 2 out]
                        n168 = property class="DigNum (strict)"(reference=w521, error in=w523, "Format & Precision:Format"=w518) -> (reference out=w524:refnum<vi>, error out=w522:errorcluster)
                        n169 = Close Reference(reference=w524) -> ()  [unwired: 1 in, 1 out]
                      }
                      frame "Format String" {
                        n170 = property class="DigNum (strict)"(reference=w526, error in=w528, "Format String"=w525) -> (reference out=w529:refnum<vi>, error out=w527:errorcluster)
                        n171 = Close Reference(reference=w529) -> ()  [unwired: 1 in, 1 out]
                      }
                      frame "Increment" {
                        n172 = Fract/Exp String To Number(string=w532, default (0 dbl)=0.0 ("Data Range:Minimum")) -> (number=w530:dbl)  [unwired: 3 out]
                        n173 = property class="DigNum (strict)"(reference=w533, error in=w535, "Data Range:Increment"=w530) -> (reference out=w536:refnum<vi>, error out=w534:errorcluster)
                        n174 = Close Reference(reference=w536) -> ()  [unwired: 1 in, 1 out]
                      }
                      frame "Maximum" {
                        n175 = Fract/Exp String To Number(string=w539, default (0 dbl)=0.0 ("Data Range:Minimum")) -> (number=w537:dbl)  [unwired: 3 out]
                        n176 = property class="DigNum (strict)"(reference=w540, error in=w542, "Data Range:Maximum"=w537) -> (reference out=w543:refnum<vi>, error out=w541:errorcluster)
                        n177 = Close Reference(reference=w543) -> ()  [unwired: 1 in, 1 out]
                      }
                      frame "Minimum" {
                        n178 = Fract/Exp String To Number(string=w546, default (0 dbl)=0.0 ("Data Range:Minimum")) -> (number=w544:dbl)  [unwired: 3 out]
                        n179 = property class="DigNum (strict)"(reference=w547, error in=w549, "Data Range:Minimum"=w544) -> (reference out=w550:refnum<vi>, error out=w548:errorcluster)
                        n180 = Close Reference(reference=w550) -> ()  [unwired: 1 in, 1 out]
                      }
                      frame "Precision" {
                        n181 = Decimal String To Number(string=w553, default (0L)=u8 0 ("Format & Precision:Format")) -> (number=w551:u8)  [unwired: 2 out]
                        n182 = property class="DigNum (strict)"(reference=w554, error in=w556, "Format & Precision:Precision"=w551) -> (reference out=w557:refnum<vi>, error out=w555:errorcluster)
                        n183 = Close Reference(reference=w557) -> ()  [unwired: 1 in, 1 out]
                      }
                      frame "Value" {
                        n184 = Empty String/Path?(string/path=w563) -> (empty?=w562:bool)
                        n185 = Not(x=w562) -> (.not. x?=w561:bool)
                        n186 = Fract/Exp String To Number(string=w563, default (0 dbl)=0.0) -> (number=w560:dbl)  [unwired: 3 out]
                        n187 = Select(t=w560, s=w561, f=nan) -> (s? t:f=w559:dbl)
                        n188 = property class="DigNum (strict)"(reference=w565, error in=w567, "Value"=w559) -> (error out=w566:errorcluster)  [unwired: 1 out]
                      }
                    }
                  }
                  frame 11 {
                    n189 = Type Cast(type=refnum<vi> refnum ("EXT"), x=w574) -> (*(type *) &x=w571:refnum<vi>)
                    n190 = case shown="\"Value\"" w572 {
                      tunnel: w570 -> [w575 w585 w591 w597 w603 w607 w613 w619]
                      tunnel: [w575 w584 w590 w596 w602 w606 w612 w618] -> w569
                      tunnel: w571 -> [_ w583 w589 w595 w601 w605 w611 w617]
                      tunnel: w568 -> [_ w578 w588 w594 w600 w604 w610 w616]
                      frame "False", Default {
                      }
                      frame "Value" {
                        n191 = Empty String/Path?(string/path=w578) -> (empty?=w581:bool)
                        n192 = Not(x=w581) -> (.not. x?=w580:bool)
                        n193 = Fract/Exp String To Number(string=w578, default (0 dbl)=ext 0.0) -> (number=w577:ext)  [unwired: 3 out]
                        n194 = Select(t=w577, s=w580, f=ext nan) -> (s? t:f=w576:ext)
                        n195 = property class="DigNum (strict)"(reference=w583, error in=w585, "Value"=w576) -> (error out=w584:errorcluster)  [unwired: 1 out]
                      }
                      frame "Minimum" {
                        n196 = Fract/Exp String To Number(string=w588, default (0 dbl)=0.0 ("Data Range:Minimum")) -> (number=w586:dbl)  [unwired: 3 out]
                        n197 = property class="DigNum (strict)"(reference=w589, error in=w591, "Data Range:Minimum"=w586) -> (error out=w590:errorcluster)  [unwired: 1 out]
                      }
                      frame "Maximum" {
                        n198 = Fract/Exp String To Number(string=w594, default (0 dbl)=0.0 ("Data Range:Minimum")) -> (number=w592:dbl)  [unwired: 3 out]
                        n199 = property class="DigNum (strict)"(reference=w595, error in=w597, "Data Range:Maximum"=w592) -> (error out=w596:errorcluster)  [unwired: 1 out]
                      }
                      frame "Increment" {
                        n200 = Fract/Exp String To Number(string=w600, default (0 dbl)=0.0 ("Data Range:Minimum")) -> (number=w598:dbl)  [unwired: 3 out]
                        n201 = property class="DigNum (strict)"(reference=w601, error in=w603, "Data Range:Increment"=w598) -> (error out=w602:errorcluster)  [unwired: 1 out]
                      }
                      frame "Format String" {
                        n202 = property class="DigNum (strict)"(reference=w605, error in=w607, "Format String"=w604) -> (error out=w606:errorcluster)  [unwired: 1 out]
                      }
                      frame "Format" {
                        n203 = Decimal String To Number(string=w610, default (0L)=u8 0 ("Format & Precision:Format")) -> (number=w608:u8)  [unwired: 2 out]
                        n204 = property class="DigNum (strict)"(reference=w611, error in=w613, "Format & Precision:Format"=w608) -> (error out=w612:errorcluster)  [unwired: 1 out]
                      }
                      frame "Precision" {
                        n205 = Decimal String To Number(string=w616, default (0L)=u8 0 ("Format & Precision:Format")) -> (number=w614:u8)  [unwired: 2 out]
                        n206 = property class="DigNum (strict)"(reference=w617, error in=w619, "Format & Precision:Precision"=w614) -> (error out=w618:errorcluster)  [unwired: 1 out]
                      }
                    }
                  }
                }
              }
              frame "Slide" {
                n207 = case shown="2" w621 {
                  tunnel: w625 -> [w626 w629 w707 w785 w863 w943 w1018 w1097 w1174 w1253]
                  tunnel: [w626 w627 w705 w783 w864 w944 w1021 w1095 w1175 w1251] -> w624
                  tunnel: w623 -> [_ w633 w711 w789 w867 w945 w1023 w1101 w1179 w1257]
                  tunnel: w622 -> [_ w628 w706 w784 w862 w940 w1017 w1096 w1173 w1252]
                  tunnel: w620 -> [_ w631 w709 w787 w866 w941 w1020 w1099 w1177 w1255]
                  frame 0, Default {
                  }
                  frame 9 {
                    n208 = Type Cast(type=refnum<vi> refnum ("Slide"), x=w633) -> (*(type *) &x=w630:refnum<vi>)
                    n209 = case shown="\"Value\"" w631 {
                      tunnel: w629 -> [w634 w640 w646 w652 w658 w664 w670 w676 w682 w688 w692 w698 w704]
                      tunnel: [w634 w639 w645 w651 w657 w663 w669 w675 w681 w687 w691 w697 w703] -> w627
                      tunnel: w630 -> [_ w638 w644 w650 w656 w662 w668 w674 w680 w686 w690 w696 w702]
                      tunnel: w628 -> [_ w637 w643 w649 w655 w661 w667 w673 w679 w685 w689 w695 w701]
                      frame "False", Default {
                      }
                      frame "Value" {
                        n210 = Fract/Exp String To Number(string=w637, default (0 dbl)=sgl 0.0) -> (number=w636:sgl)  [unwired: 3 out]
                        n211 = property class="Slide (strict)"(reference=w638, error in=w640, "Value"=w636) -> (error out=w639:errorcluster)  [unwired: 1 out]
                      }
                      frame "Minimum" {
                        n212 = Fract/Exp String To Number(string=w643, default (0 dbl)=0.0 ("Data Range:Minimum")) -> (number=w641:dbl)  [unwired: 3 out]
                        n213 = property class="Slide (strict)"(reference=w644, error in=w646, "Data Range:Minimum"=w641) -> (error out=w645:errorcluster)  [unwired: 1 out]
                      }
                      frame "Scale.Minimum" {
                        n214 = Fract/Exp String To Number(string=w649, default (0 dbl)=0.0 ("Data Range:Minimum")) -> (number=w647:dbl)  [unwired: 3 out]
                        n215 = property class="Slide (strict)"(reference=w650, error in=w652, "Scale.Range:Minimum"=w647) -> (error out=w651:errorcluster)  [unwired: 1 out]
                      }
                      frame "Maximum" {
                        n216 = Fract/Exp String To Number(string=w655, default (0 dbl)=0.0 ("Data Range:Minimum")) -> (number=w653:dbl)  [unwired: 3 out]
                        n217 = property class="Slide (strict)"(reference=w656, error in=w658, "Data Range:Maximum"=w653) -> (error out=w657:errorcluster)  [unwired: 1 out]
                      }
                      frame "Scale.Maximum" {
                        n218 = Fract/Exp String To Number(string=w661, default (0 dbl)=0.0 ("Data Range:Minimum")) -> (number=w659:dbl)  [unwired: 3 out]
                        n219 = property class="Slide (strict)"(reference=w662, error in=w664, "Scale.Range:Maximum"=w659) -> (error out=w663:errorcluster)  [unwired: 1 out]
                      }
                      frame "Increment" {
                        n220 = Fract/Exp String To Number(string=w667, default (0 dbl)=0.0 ("Data Range:Minimum")) -> (number=w665:dbl)  [unwired: 3 out]
                        n221 = property class="Slide (strict)"(reference=w668, error in=w670, "Data Range:Increment"=w665) -> (error out=w669:errorcluster)  [unwired: 1 out]
                      }
                      frame "Scale.Increment" {
                        n222 = Fract/Exp String To Number(string=w673, default (0 dbl)=0.0 ("Data Range:Minimum")) -> (number=w671:dbl)  [unwired: 3 out]
                        n223 = property class="Slide (strict)"(reference=w674, error in=w676, "Scale.Range:Increment"=w671) -> (error out=w675:errorcluster)  [unwired: 1 out]
                      }
                      frame "Scale.Start" {
                        n224 = Fract/Exp String To Number(string=w679, default (0 dbl)=0.0 ("Data Range:Minimum")) -> (number=w677:dbl)  [unwired: 3 out]
                        n225 = property class="Slide (strict)"(reference=w680, error in=w682, "Scale.Range:Start"=w677) -> (error out=w681:errorcluster)  [unwired: 1 out]
                      }
                      frame "Scale.MinorInc" {
                        n226 = Fract/Exp String To Number(string=w685, default (0 dbl)=0.0 ("Data Range:Minimum")) -> (number=w683:dbl)  [unwired: 3 out]
                        n227 = property class="Slide (strict)"(reference=w686, error in=w688, "Scale.Range:Minor Increment"=w683) -> (error out=w687:errorcluster)  [unwired: 1 out]
                      }
                      frame "Scale.Format String" {
                        n228 = property class="Slide (strict)"(reference=w690, error in=w692, "Scale.Format String"=w689) -> (error out=w691:errorcluster)  [unwired: 1 out]
                      }
                      frame "Scale.Format" {
                        n229 = Decimal String To Number(string=w695, default (0L)=u8 0 ("Format & Precision:Format")) -> (number=w693:u8)  [unwired: 2 out]
                        n230 = property class="Slide (strict)"(reference=w696, error in=w698, "Scale.Format & Precision:Format"=w693) -> (error out=w697:errorcluster)  [unwired: 1 out]
                      }
                      frame "Scale.Precision" {
                        n231 = Decimal String To Number(string=w701, default (0L)=u8 0 ("Format & Precision:Format")) -> (number=w699:u8)  [unwired: 2 out]
                        n232 = property class="Slide (strict)"(reference=w702, error in=w704, "Scale.Format & Precision:Precision"=w699) -> (error out=w703:errorcluster)  [unwired: 1 out]
                      }
                    }
                  }
                  frame 10 {
                    n233 = Type Cast(type=refnum<vi> refnum ("Slide"), x=w711) -> (*(type *) &x=w708:refnum<vi>)
                    n234 = case shown="\"Value\"" w709 {
                      tunnel: w707 -> [w712 w718 w724 w730 w736 w742 w748 w754 w760 w766 w770 w776 w782]
                      tunnel: [w712 w717 w723 w729 w735 w741 w747 w753 w759 w765 w769 w775 w781] -> w705
                      tunnel: w708 -> [_ w716 w722 w728 w734 w740 w746 w752 w758 w764 w768 w774 w780]
                      tunnel: w706 -> [_ w715 w721 w727 w733 w739 w745 w751 w757 w763 w767 w773 w779]
                      frame "False", Default {
                      }
                      frame "Value" {
                        n235 = Fract/Exp String To Number(string=w715, default (0 dbl)=0.0) -> (number=w714:dbl)  [unwired: 3 out]
                        n236 = property class="Slide (strict)"(reference=w716, error in=w718, "Value"=w714) -> (error out=w717:errorcluster)  [unwired: 1 out]
                      }
                      frame "Minimum" {
                        n237 = Fract/Exp String To Number(string=w721, default (0 dbl)=0.0 ("Data Range:Minimum")) -> (number=w719:dbl)  [unwired: 3 out]
                        n238 = property class="Slide (strict)"(reference=w722, error in=w724, "Data Range:Minimum"=w719) -> (error out=w723:errorcluster)  [unwired: 1 out]
                      }
                      frame "Scale.Minimum" {
                        n239 = Fract/Exp String To Number(string=w727, default (0 dbl)=0.0 ("Data Range:Minimum")) -> (number=w725:dbl)  [unwired: 3 out]
                        n240 = property class="Slide (strict)"(reference=w728, error in=w730, "Scale.Range:Minimum"=w725) -> (error out=w729:errorcluster)  [unwired: 1 out]
                      }
                      frame "Maximum" {
                        n241 = Fract/Exp String To Number(string=w733, default (0 dbl)=0.0 ("Data Range:Minimum")) -> (number=w731:dbl)  [unwired: 3 out]
                        n242 = property class="Slide (strict)"(reference=w734, error in=w736, "Data Range:Maximum"=w731) -> (error out=w735:errorcluster)  [unwired: 1 out]
                      }
                      frame "Scale.Maximum" {
                        n243 = Fract/Exp String To Number(string=w739, default (0 dbl)=0.0 ("Data Range:Minimum")) -> (number=w737:dbl)  [unwired: 3 out]
                        n244 = property class="Slide (strict)"(reference=w740, error in=w742, "Scale.Range:Maximum"=w737) -> (error out=w741:errorcluster)  [unwired: 1 out]
                      }
                      frame "Increment" {
                        n245 = Fract/Exp String To Number(string=w745, default (0 dbl)=0.0 ("Data Range:Minimum")) -> (number=w743:dbl)  [unwired: 3 out]
                        n246 = property class="Slide (strict)"(reference=w746, error in=w748, "Data Range:Increment"=w743) -> (error out=w747:errorcluster)  [unwired: 1 out]
                      }
                      frame "Scale.Increment" {
                        n247 = Fract/Exp String To Number(string=w751, default (0 dbl)=0.0 ("Data Range:Minimum")) -> (number=w749:dbl)  [unwired: 3 out]
                        n248 = property class="Slide (strict)"(reference=w752, error in=w754, "Scale.Range:Increment"=w749) -> (error out=w753:errorcluster)  [unwired: 1 out]
                      }
                      frame "Scale.Start" {
                        n249 = Fract/Exp String To Number(string=w757, default (0 dbl)=0.0 ("Data Range:Minimum")) -> (number=w755:dbl)  [unwired: 3 out]
                        n250 = property class="Slide (strict)"(reference=w758, error in=w760, "Scale.Range:Start"=w755) -> (error out=w759:errorcluster)  [unwired: 1 out]
                      }
                      frame "Scale.MinorInc" {
                        n251 = Fract/Exp String To Number(string=w763, default (0 dbl)=0.0 ("Data Range:Minimum")) -> (number=w761:dbl)  [unwired: 3 out]
                        n252 = property class="Slide (strict)"(reference=w764, error in=w766, "Scale.Range:Minor Increment"=w761) -> (error out=w765:errorcluster)  [unwired: 1 out]
                      }
                      frame "Scale.Format String" {
                        n253 = property class="Slide (strict)"(reference=w768, error in=w770, "Scale.Format String"=w767) -> (error out=w769:errorcluster)  [unwired: 1 out]
                      }
                      frame "Scale.Format" {
                        n254 = Decimal String To Number(string=w773, default (0L)=u8 0 ("Format & Precision:Format")) -> (number=w771:u8)  [unwired: 2 out]
                        n255 = property class="Slide (strict)"(reference=w774, error in=w776, "Scale.Format & Precision:Format"=w771) -> (error out=w775:errorcluster)  [unwired: 1 out]
                      }
                      frame "Scale.Precision" {
                        n256 = Decimal String To Number(string=w779, default (0L)=u8 0 ("Format & Precision:Format")) -> (number=w777:u8)  [unwired: 2 out]
                        n257 = property class="Slide (strict)"(reference=w780, error in=w782, "Scale.Format & Precision:Precision"=w777) -> (error out=w781:errorcluster)  [unwired: 1 out]
                      }
                    }
                  }
                  frame 11 {
                    n258 = Type Cast(type=refnum<vi> refnum ("Slide"), x=w789) -> (*(type *) &x=w786:refnum<vi>)
                    n259 = case shown="\"Value\"" w787 {
                      tunnel: w785 -> [w790 w796 w802 w808 w814 w820 w826 w832 w838 w844 w848 w854 w860]
                      tunnel: [w790 w795 w801 w807 w813 w819 w825 w831 w837 w843 w847 w853 w859] -> w783
                      tunnel: w786 -> [_ w794 w800 w806 w812 w818 w824 w830 w836 w842 w846 w852 w858]
                      tunnel: w784 -> [_ w793 w799 w805 w811 w817 w823 w829 w835 w841 w845 w851 w857]
                      frame "False", Default {
                      }
                      frame "Value" {
                        n260 = Fract/Exp String To Number(string=w793, default (0 dbl)=ext 0.0) -> (number=w792:ext)  [unwired: 3 out]
                        n261 = property class="Slide (strict)"(reference=w794, error in=w796, "Value"=w792) -> (error out=w795:errorcluster)  [unwired: 1 out]
                      }
                      frame "Minimum" {
                        n262 = Fract/Exp String To Number(string=w799, default (0 dbl)=0.0 ("Data Range:Minimum")) -> (number=w797:dbl)  [unwired: 3 out]
                        n263 = property class="Slide (strict)"(reference=w800, error in=w802, "Data Range:Minimum"=w797) -> (error out=w801:errorcluster)  [unwired: 1 out]
                      }
                      frame "Scale.Minimum" {
                        n264 = Fract/Exp String To Number(string=w805, default (0 dbl)=0.0 ("Data Range:Minimum")) -> (number=w803:dbl)  [unwired: 3 out]
                        n265 = property class="Slide (strict)"(reference=w806, error in=w808, "Scale.Range:Minimum"=w803) -> (error out=w807:errorcluster)  [unwired: 1 out]
                      }
                      frame "Maximum" {
                        n266 = Fract/Exp String To Number(string=w811, default (0 dbl)=0.0 ("Data Range:Minimum")) -> (number=w809:dbl)  [unwired: 3 out]
                        n267 = property class="Slide (strict)"(reference=w812, error in=w814, "Data Range:Maximum"=w809) -> (error out=w813:errorcluster)  [unwired: 1 out]
                      }
                      frame "Scale.Maximum" {
                        n268 = Fract/Exp String To Number(string=w817, default (0 dbl)=0.0 ("Data Range:Minimum")) -> (number=w815:dbl)  [unwired: 3 out]
                        n269 = property class="Slide (strict)"(reference=w818, error in=w820, "Scale.Range:Maximum"=w815) -> (error out=w819:errorcluster)  [unwired: 1 out]
                      }
                      frame "Increment" {
                        n270 = Fract/Exp String To Number(string=w823, default (0 dbl)=0.0 ("Data Range:Minimum")) -> (number=w821:dbl)  [unwired: 3 out]
                        n271 = property class="Slide (strict)"(reference=w824, error in=w826, "Data Range:Increment"=w821) -> (error out=w825:errorcluster)  [unwired: 1 out]
                      }
                      frame "Scale.Increment" {
                        n272 = Fract/Exp String To Number(string=w829, default (0 dbl)=0.0 ("Data Range:Minimum")) -> (number=w827:dbl)  [unwired: 3 out]
                        n273 = property class="Slide (strict)"(reference=w830, error in=w832, "Scale.Range:Increment"=w827) -> (error out=w831:errorcluster)  [unwired: 1 out]
                      }
                      frame "Scale.Start" {
                        n274 = Fract/Exp String To Number(string=w835, default (0 dbl)=0.0 ("Data Range:Minimum")) -> (number=w833:dbl)  [unwired: 3 out]
                        n275 = property class="Slide (strict)"(reference=w836, error in=w838, "Scale.Range:Start"=w833) -> (error out=w837:errorcluster)  [unwired: 1 out]
                      }
                      frame "Scale.MinorInc" {
                        n276 = Fract/Exp String To Number(string=w841, default (0 dbl)=0.0 ("Data Range:Minimum")) -> (number=w839:dbl)  [unwired: 3 out]
                        n277 = property class="Slide (strict)"(reference=w842, error in=w844, "Scale.Range:Minor Increment"=w839) -> (error out=w843:errorcluster)  [unwired: 1 out]
                      }
                      frame "Scale.Format String" {
                        n278 = property class="Slide (strict)"(reference=w846, error in=w848, "Scale.Format String"=w845) -> (error out=w847:errorcluster)  [unwired: 1 out]
                      }
                      frame "Scale.Format" {
                        n279 = Decimal String To Number(string=w851, default (0L)=u8 0 ("Format & Precision:Format")) -> (number=w849:u8)  [unwired: 2 out]
                        n280 = property class="Slide (strict)"(reference=w852, error in=w854, "Scale.Format & Precision:Format"=w849) -> (error out=w853:errorcluster)  [unwired: 1 out]
                      }
                      frame "Scale.Precision" {
                        n281 = Decimal String To Number(string=w857, default (0L)=u8 0 ("Format & Precision:Format")) -> (number=w855:u8)  [unwired: 2 out]
                        n282 = property class="Slide (strict)"(reference=w858, error in=w860, "Scale.Format & Precision:Precision"=w855) -> (error out=w859:errorcluster)  [unwired: 1 out]
                      }
                    }
                  }
                  frame 1 {
                    n283 = Type Cast(type=refnum<vi> refnum ("Slide"), x=w867) -> (*(type *) &x=w865:refnum<vi>)
                    n284 = case shown="\"Value\"" w866 {
                      tunnel: w863 -> [w868 w874 w880 w886 w892 w898 w904 w910 w916 w922 w926 w932 w938]
                      tunnel: [w868 w873 w879 w885 w891 w897 w903 w909 w915 w921 w925 w931 w937] -> w864
                      tunnel: w865 -> [_ w872 w878 w884 w890 w896 w902 w908 w914 w920 w924 w930 w936]
                      tunnel: w862 -> [_ w871 w877 w883 w889 w895 w901 w907 w913 w919 w923 w929 w935]
                      frame "False", Default {
                      }
                      frame "Value" {
                        n285 = Fract/Exp String To Number(string=w871, default (0 dbl)=u8 0) -> (number=w870:u8)  [unwired: 3 out]
                        n286 = property class="Slide (strict)"(reference=w872, error in=w874, "Value"=w870) -> (error out=w873:errorcluster)  [unwired: 1 out]
                      }
                      frame "Minimum" {
                        n287 = Fract/Exp String To Number(string=w877, default (0 dbl)=0.0 ("Data Range:Minimum")) -> (number=w875:dbl)  [unwired: 3 out]
                        n288 = property class="Slide (strict)"(reference=w878, error in=w880, "Data Range:Minimum"=w875) -> (error out=w879:errorcluster)  [unwired: 1 out]
                      }
                      frame "Scale.Minimum" {
                        n289 = Fract/Exp String To Number(string=w883, default (0 dbl)=0.0 ("Data Range:Minimum")) -> (number=w881:dbl)  [unwired: 3 out]
                        n290 = property class="Slide (strict)"(reference=w884, error in=w886, "Scale.Range:Minimum"=w881) -> (error out=w885:errorcluster)  [unwired: 1 out]
                      }
                      frame "Maximum" {
                        n291 = Fract/Exp String To Number(string=w889, default (0 dbl)=0.0 ("Data Range:Minimum")) -> (number=w887:dbl)  [unwired: 3 out]
                        n292 = property class="Slide (strict)"(reference=w890, error in=w892, "Data Range:Maximum"=w887) -> (error out=w891:errorcluster)  [unwired: 1 out]
                      }
                      frame "Scale.Maximum" {
                        n293 = Fract/Exp String To Number(string=w895, default (0 dbl)=0.0 ("Data Range:Minimum")) -> (number=w893:dbl)  [unwired: 3 out]
                        n294 = property class="Slide (strict)"(reference=w896, error in=w898, "Scale.Range:Maximum"=w893) -> (error out=w897:errorcluster)  [unwired: 1 out]
                      }
                      frame "Increment" {
                        n295 = Fract/Exp String To Number(string=w901, default (0 dbl)=0.0 ("Data Range:Minimum")) -> (number=w899:dbl)  [unwired: 3 out]
                        n296 = property class="Slide (strict)"(reference=w902, error in=w904, "Data Range:Increment"=w899) -> (error out=w903:errorcluster)  [unwired: 1 out]
                      }
                      frame "Scale.Increment" {
                        n297 = Fract/Exp String To Number(string=w907, default (0 dbl)=0.0 ("Data Range:Minimum")) -> (number=w905:dbl)  [unwired: 3 out]
                        n298 = property class="Slide (strict)"(reference=w908, error in=w910, "Scale.Range:Increment"=w905) -> (error out=w909:errorcluster)  [unwired: 1 out]
                      }
                      frame "Scale.Start" {
                        n299 = Fract/Exp String To Number(string=w913, default (0 dbl)=0.0 ("Data Range:Minimum")) -> (number=w911:dbl)  [unwired: 3 out]
                        n300 = property class="Slide (strict)"(reference=w914, error in=w916, "Scale.Range:Start"=w911) -> (error out=w915:errorcluster)  [unwired: 1 out]
                      }
                      frame "Scale.MinorInc" {
                        n301 = Fract/Exp String To Number(string=w919, default (0 dbl)=0.0 ("Data Range:Minimum")) -> (number=w917:dbl)  [unwired: 3 out]
                        n302 = property class="Slide (strict)"(reference=w920, error in=w922, "Scale.Range:Minor Increment"=w917) -> (error out=w921:errorcluster)  [unwired: 1 out]
                      }
                      frame "Scale.Format String" {
                        n303 = property class="Slide (strict)"(reference=w924, error in=w926, "Scale.Format String"=w923) -> (error out=w925:errorcluster)  [unwired: 1 out]
                      }
                      frame "Scale.Format" {
                        n304 = Decimal String To Number(string=w929, default (0L)=u8 0 ("Format & Precision:Format")) -> (number=w927:u8)  [unwired: 2 out]
                        n305 = property class="Slide (strict)"(reference=w930, error in=w932, "Scale.Format & Precision:Format"=w927) -> (error out=w931:errorcluster)  [unwired: 1 out]
                      }
                      frame "Scale.Precision" {
                        n306 = Decimal String To Number(string=w935, default (0L)=u8 0 ("Format & Precision:Format")) -> (number=w933:u8)  [unwired: 2 out]
                        n307 = property class="Slide (strict)"(reference=w936, error in=w938, "Scale.Format & Precision:Precision"=w933) -> (error out=w937:errorcluster)  [unwired: 1 out]
                      }
                    }
                  }
                  frame 2 {
                    n308 = Type Cast(type=refnum<vi> refnum ("Slide"), x=w945) -> (*(type *) &x=w942:refnum<vi>)
                    n309 = case shown="\"Value\"" w941 {
                      tunnel: w943 -> [w946 w952 w958 w964 w970 w976 w982 w988 w994 w1000 w1004 w1010 w1016]
                      tunnel: [w946 w951 w957 w963 w969 w975 w981 w987 w993 w999 w1003 w1009 w1015] -> w944
                      tunnel: w942 -> [_ w950 w956 w962 w968 w974 w980 w986 w992 w998 w1002 w1008 w1014]
                      tunnel: w940 -> [_ w949 w955 w961 w967 w973 w979 w985 w991 w997 w1001 w1007 w1013]
                      frame "False", Default {
                      }
                      frame "Value" {
                        n310 = Fract/Exp String To Number(string=w949, default (0 dbl)=u16 0) -> (number=w948:u16)  [unwired: 3 out]
                        n311 = property class="Slide (strict)"(reference=w950, error in=w952, "Value"=w948) -> (error out=w951:errorcluster)  [unwired: 1 out]
                      }
                      frame "Minimum" {
                        n312 = Fract/Exp String To Number(string=w955, default (0 dbl)=0.0 ("Data Range:Minimum")) -> (number=w953:dbl)  [unwired: 3 out]
                        n313 = property class="Slide (strict)"(reference=w956, error in=w958, "Data Range:Minimum"=w953) -> (error out=w957:errorcluster)  [unwired: 1 out]
                      }
                      frame "Scale.Minimum" {
                        n314 = Fract/Exp String To Number(string=w961, default (0 dbl)=0.0 ("Data Range:Minimum")) -> (number=w959:dbl)  [unwired: 3 out]
                        n315 = property class="Slide (strict)"(reference=w962, error in=w964, "Scale.Range:Minimum"=w959) -> (error out=w963:errorcluster)  [unwired: 1 out]
                      }
                      frame "Maximum" {
                        n316 = Fract/Exp String To Number(string=w967, default (0 dbl)=0.0 ("Data Range:Minimum")) -> (number=w965:dbl)  [unwired: 3 out]
                        n317 = property class="Slide (strict)"(reference=w968, error in=w970, "Data Range:Maximum"=w965) -> (error out=w969:errorcluster)  [unwired: 1 out]
                      }
                      frame "Scale.Maximum" {
                        n318 = Fract/Exp String To Number(string=w973, default (0 dbl)=0.0 ("Data Range:Minimum")) -> (number=w971:dbl)  [unwired: 3 out]
                        n319 = property class="Slide (strict)"(reference=w974, error in=w976, "Scale.Range:Maximum"=w971) -> (error out=w975:errorcluster)  [unwired: 1 out]
                      }
                      frame "Increment" {
                        n320 = Fract/Exp String To Number(string=w979, default (0 dbl)=0.0 ("Data Range:Minimum")) -> (number=w977:dbl)  [unwired: 3 out]
                        n321 = property class="Slide (strict)"(reference=w980, error in=w982, "Data Range:Increment"=w977) -> (error out=w981:errorcluster)  [unwired: 1 out]
                      }
                      frame "Scale.Increment" {
                        n322 = Fract/Exp String To Number(string=w985, default (0 dbl)=0.0 ("Data Range:Minimum")) -> (number=w983:dbl)  [unwired: 3 out]
                        n323 = property class="Slide (strict)"(reference=w986, error in=w988, "Scale.Range:Increment"=w983) -> (error out=w987:errorcluster)  [unwired: 1 out]
                      }
                      frame "Scale.Start" {
                        n324 = Fract/Exp String To Number(string=w991, default (0 dbl)=0.0 ("Data Range:Minimum")) -> (number=w989:dbl)  [unwired: 3 out]
                        n325 = property class="Slide (strict)"(reference=w992, error in=w994, "Scale.Range:Start"=w989) -> (error out=w993:errorcluster)  [unwired: 1 out]
                      }
                      frame "Scale.MinorInc" {
                        n326 = Fract/Exp String To Number(string=w997, default (0 dbl)=0.0 ("Data Range:Minimum")) -> (number=w995:dbl)  [unwired: 3 out]
                        n327 = property class="Slide (strict)"(reference=w998, error in=w1000, "Scale.Range:Minor Increment"=w995) -> (error out=w999:errorcluster)  [unwired: 1 out]
                      }
                      frame "Scale.Format String" {
                        n328 = property class="Slide (strict)"(reference=w1002, error in=w1004, "Scale.Format String"=w1001) -> (error out=w1003:errorcluster)  [unwired: 1 out]
                      }
                      frame "Scale.Format" {
                        n329 = Decimal String To Number(string=w1007, default (0L)=u8 0 ("Format & Precision:Format")) -> (number=w1005:u8)  [unwired: 2 out]
                        n330 = property class="Slide (strict)"(reference=w1008, error in=w1010, "Scale.Format & Precision:Format"=w1005) -> (error out=w1009:errorcluster)  [unwired: 1 out]
                      }
                      frame "Scale.Precision" {
                        n331 = Decimal String To Number(string=w1013, default (0L)=u8 0 ("Format & Precision:Format")) -> (number=w1011:u8)  [unwired: 2 out]
                        n332 = property class="Slide (strict)"(reference=w1014, error in=w1016, "Scale.Format & Precision:Precision"=w1011) -> (error out=w1015:errorcluster)  [unwired: 1 out]
                      }
                    }
                  }
                  frame 3 {
                    n333 = Type Cast(type=refnum<vi> refnum ("Slide"), x=w1023) -> (*(type *) &x=w1019:refnum<vi>)
                    n334 = case shown="\"Value\"" w1020 {
                      tunnel: [w1024 w1030 w1036 w1042 w1048 w1054 w1060 w1066 w1072 w1078 w1082 w1088 w1094] -> w1021
                      tunnel: w1019 -> [_ w1025 w1031 w1039 w1044 w1050 w1056 w1062 w1067 w1075 w1080 w1083 w1091]
                      tunnel: w1018 -> [w1024 w1027 w1033 w1038 w1043 w1051 w1057 w1063 w1069 w1074 w1081 w1085 w1089]
                      tunnel: w1017 -> [_ w1026 w1032 w1037 w1045 w1049 w1055 w1061 w1068 w1073 w1079 w1084 w1090]
                      frame "False", Default {
                      }
                      frame "Value" {
                        n335 = Fract/Exp String To Number(string=w1026, default (0 dbl)=0) -> (number=w1029:i32)  [unwired: 3 out]
                        n336 = property class="Slide (strict)"(reference=w1025, error in=w1027, "Value"=w1029) -> (error out=w1030:errorcluster)  [unwired: 1 out]
                      }
                      frame "Minimum" {
                        n337 = Fract/Exp String To Number(string=w1032, default (0 dbl)=0.0 ("Data Range:Minimum")) -> (number=w1034:dbl)  [unwired: 3 out]
                        n338 = property class="Slide (strict)"(reference=w1031, error in=w1033, "Data Range:Minimum"=w1034) -> (error out=w1036:errorcluster)  [unwired: 1 out]
                      }
                      frame "Scale.Minimum" {
                        n339 = Fract/Exp String To Number(string=w1037, default (0 dbl)=0.0 ("Data Range:Minimum")) -> (number=w1040:dbl)  [unwired: 3 out]
                        n340 = property class="Slide (strict)"(reference=w1039, error in=w1038, "Scale.Range:Minimum"=w1040) -> (error out=w1042:errorcluster)  [unwired: 1 out]
                      }
                      frame "Maximum" {
                        n341 = Fract/Exp String To Number(string=w1045, default (0 dbl)=0.0 ("Data Range:Minimum")) -> (number=w1046:dbl)  [unwired: 3 out]
                        n342 = property class="Slide (strict)"(reference=w1044, error in=w1043, "Data Range:Maximum"=w1046) -> (error out=w1048:errorcluster)  [unwired: 1 out]
                      }
                      frame "Scale.Maximum" {
                        n343 = Fract/Exp String To Number(string=w1049, default (0 dbl)=0.0 ("Data Range:Minimum")) -> (number=w1052:dbl)  [unwired: 3 out]
                        n344 = property class="Slide (strict)"(reference=w1050, error in=w1051, "Scale.Range:Maximum"=w1052) -> (error out=w1054:errorcluster)  [unwired: 1 out]
                      }
                      frame "Increment" {
                        n345 = Fract/Exp String To Number(string=w1055, default (0 dbl)=0.0 ("Data Range:Minimum")) -> (number=w1058:dbl)  [unwired: 3 out]
                        n346 = property class="Slide (strict)"(reference=w1056, error in=w1057, "Data Range:Increment"=w1058) -> (error out=w1060:errorcluster)  [unwired: 1 out]
                      }
                      frame "Scale.Increment" {
                        n347 = Fract/Exp String To Number(string=w1061, default (0 dbl)=0.0 ("Data Range:Minimum")) -> (number=w1064:dbl)  [unwired: 3 out]
                        n348 = property class="Slide (strict)"(reference=w1062, error in=w1063, "Scale.Range:Increment"=w1064) -> (error out=w1066:errorcluster)  [unwired: 1 out]
                      }
                      frame "Scale.Start" {
                        n349 = Fract/Exp String To Number(string=w1068, default (0 dbl)=0.0 ("Data Range:Minimum")) -> (number=w1070:dbl)  [unwired: 3 out]
                        n350 = property class="Slide (strict)"(reference=w1067, error in=w1069, "Scale.Range:Start"=w1070) -> (error out=w1072:errorcluster)  [unwired: 1 out]
                      }
                      frame "Scale.MinorInc" {
                        n351 = Fract/Exp String To Number(string=w1073, default (0 dbl)=0.0 ("Data Range:Minimum")) -> (number=w1076:dbl)  [unwired: 3 out]
                        n352 = property class="Slide (strict)"(reference=w1075, error in=w1074, "Scale.Range:Minor Increment"=w1076) -> (error out=w1078:errorcluster)  [unwired: 1 out]
                      }
                      frame "Scale.Format String" {
                        n353 = property class="Slide (strict)"(reference=w1080, error in=w1081, "Scale.Format String"=w1079) -> (error out=w1082:errorcluster)  [unwired: 1 out]
                      }
                      frame "Scale.Format" {
                        n354 = Decimal String To Number(string=w1084, default (0L)=u8 0 ("Format & Precision:Format")) -> (number=w1086:u8)  [unwired: 2 out]
                        n355 = property class="Slide (strict)"(reference=w1083, error in=w1085, "Scale.Format & Precision:Format"=w1086) -> (error out=w1088:errorcluster)  [unwired: 1 out]
                      }
                      frame "Scale.Precision" {
                        n356 = Decimal String To Number(string=w1090, default (0L)=u8 0 ("Format & Precision:Format")) -> (number=w1092:u8)  [unwired: 2 out]
                        n357 = property class="Slide (strict)"(reference=w1091, error in=w1089, "Scale.Format & Precision:Precision"=w1092) -> (error out=w1094:errorcluster)  [unwired: 1 out]
                      }
                    }
                  }
                  frame 5 {
                    n358 = Type Cast(type=refnum<vi> refnum ("Slide"), x=w1101) -> (*(type *) &x=w1098:refnum<vi>)
                    n359 = case shown="\"Value\"" w1099 {
                      tunnel: [w1102 w1108 w1114 w1120 w1126 w1132 w1138 w1144 w1150 w1156 w1160 w1166 w1172] -> w1095
                      tunnel: w1098 -> [_ w1103 w1109 w1117 w1122 w1128 w1134 w1140 w1145 w1153 w1158 w1161 w1169]
                      tunnel: w1097 -> [w1102 w1105 w1111 w1116 w1121 w1129 w1135 w1141 w1147 w1152 w1159 w1163 w1167]
                      tunnel: w1096 -> [_ w1104 w1110 w1115 w1123 w1127 w1133 w1139 w1146 w1151 w1157 w1162 w1168]
                      frame "False", Default {
                      }
                      frame "Value" {
                        n360 = Fract/Exp String To Number(string=w1104, default (0 dbl)=u8 0) -> (number=w1107:u8)  [unwired: 3 out]
                        n361 = property class="Slide (strict)"(reference=w1103, error in=w1105, "Value"=w1107) -> (error out=w1108:errorcluster)  [unwired: 1 out]
                      }
                      frame "Minimum" {
                        n362 = Fract/Exp String To Number(string=w1110, default (0 dbl)=0.0 ("Data Range:Minimum")) -> (number=w1112:dbl)  [unwired: 3 out]
                        n363 = property class="Slide (strict)"(reference=w1109, error in=w1111, "Data Range:Minimum"=w1112) -> (error out=w1114:errorcluster)  [unwired: 1 out]
                      }
                      frame "Scale.Minimum" {
                        n364 = Fract/Exp String To Number(string=w1115, default (0 dbl)=0.0 ("Data Range:Minimum")) -> (number=w1118:dbl)  [unwired: 3 out]
                        n365 = property class="Slide (strict)"(reference=w1117, error in=w1116, "Scale.Range:Minimum"=w1118) -> (error out=w1120:errorcluster)  [unwired: 1 out]
                      }
                      frame "Maximum" {
                        n366 = Fract/Exp String To Number(string=w1123, default (0 dbl)=0.0 ("Data Range:Minimum")) -> (number=w1124:dbl)  [unwired: 3 out]
                        n367 = property class="Slide (strict)"(reference=w1122, error in=w1121, "Data Range:Maximum"=w1124) -> (error out=w1126:errorcluster)  [unwired: 1 out]
                      }
                      frame "Scale.Maximum" {
                        n368 = Fract/Exp String To Number(string=w1127, default (0 dbl)=0.0 ("Data Range:Minimum")) -> (number=w1130:dbl)  [unwired: 3 out]
                        n369 = property class="Slide (strict)"(reference=w1128, error in=w1129, "Scale.Range:Maximum"=w1130) -> (error out=w1132:errorcluster)  [unwired: 1 out]
                      }
                      frame "Increment" {
                        n370 = Fract/Exp String To Number(string=w1133, default (0 dbl)=0.0 ("Data Range:Minimum")) -> (number=w1136:dbl)  [unwired: 3 out]
                        n371 = property class="Slide (strict)"(reference=w1134, error in=w1135, "Data Range:Increment"=w1136) -> (error out=w1138:errorcluster)  [unwired: 1 out]
                      }
                      frame "Scale.Increment" {
                        n372 = Fract/Exp String To Number(string=w1139, default (0 dbl)=0.0 ("Data Range:Minimum")) -> (number=w1142:dbl)  [unwired: 3 out]
                        n373 = property class="Slide (strict)"(reference=w1140, error in=w1141, "Scale.Range:Increment"=w1142) -> (error out=w1144:errorcluster)  [unwired: 1 out]
                      }
                      frame "Scale.Start" {
                        n374 = Fract/Exp String To Number(string=w1146, default (0 dbl)=0.0 ("Data Range:Minimum")) -> (number=w1148:dbl)  [unwired: 3 out]
                        n375 = property class="Slide (strict)"(reference=w1145, error in=w1147, "Scale.Range:Start"=w1148) -> (error out=w1150:errorcluster)  [unwired: 1 out]
                      }
                      frame "Scale.MinorInc" {
                        n376 = Fract/Exp String To Number(string=w1151, default (0 dbl)=0.0 ("Data Range:Minimum")) -> (number=w1154:dbl)  [unwired: 3 out]
                        n377 = property class="Slide (strict)"(reference=w1153, error in=w1152, "Scale.Range:Minor Increment"=w1154) -> (error out=w1156:errorcluster)  [unwired: 1 out]
                      }
                      frame "Scale.Format String" {
                        n378 = property class="Slide (strict)"(reference=w1158, error in=w1159, "Scale.Format String"=w1157) -> (error out=w1160:errorcluster)  [unwired: 1 out]
                      }
                      frame "Scale.Format" {
                        n379 = Decimal String To Number(string=w1162, default (0L)=u8 0 ("Format & Precision:Format")) -> (number=w1164:u8)  [unwired: 2 out]
                        n380 = property class="Slide (strict)"(reference=w1161, error in=w1163, "Scale.Format & Precision:Format"=w1164) -> (error out=w1166:errorcluster)  [unwired: 1 out]
                      }
                      frame "Scale.Precision" {
                        n381 = Decimal String To Number(string=w1168, default (0L)=u8 0 ("Format & Precision:Format")) -> (number=w1170:u8)  [unwired: 2 out]
                        n382 = property class="Slide (strict)"(reference=w1169, error in=w1167, "Scale.Format & Precision:Precision"=w1170) -> (error out=w1172:errorcluster)  [unwired: 1 out]
                      }
                    }
                  }
                  frame 6 {
                    n383 = Type Cast(type=refnum<vi> refnum ("Slide"), x=w1179) -> (*(type *) &x=w1176:refnum<vi>)
                    n384 = case shown="\"Value\"" w1177 {
                      tunnel: [w1180 w1186 w1192 w1198 w1204 w1210 w1216 w1222 w1228 w1234 w1238 w1244 w1250] -> w1175
                      tunnel: w1176 -> [_ w1181 w1187 w1195 w1200 w1206 w1212 w1218 w1223 w1231 w1236 w1239 w1247]
                      tunnel: w1174 -> [w1180 w1183 w1189 w1194 w1199 w1207 w1213 w1219 w1225 w1230 w1237 w1241 w1245]
                      tunnel: w1173 -> [_ w1182 w1188 w1193 w1201 w1205 w1211 w1217 w1224 w1229 w1235 w1240 w1246]
                      frame "False", Default {
                      }
                      frame "Value" {
                        n385 = Fract/Exp String To Number(string=w1182, default (0 dbl)=u16 0) -> (number=w1185:u16)  [unwired: 3 out]
                        n386 = property class="Slide (strict)"(reference=w1181, error in=w1183, "Value"=w1185) -> (error out=w1186:errorcluster)  [unwired: 1 out]
                      }
                      frame "Minimum" {
                        n387 = Fract/Exp String To Number(string=w1188, default (0 dbl)=0.0 ("Data Range:Minimum")) -> (number=w1190:dbl)  [unwired: 3 out]
                        n388 = property class="Slide (strict)"(reference=w1187, error in=w1189, "Data Range:Minimum"=w1190) -> (error out=w1192:errorcluster)  [unwired: 1 out]
                      }
                      frame "Scale.Minimum" {
                        n389 = Fract/Exp String To Number(string=w1193, default (0 dbl)=0.0 ("Data Range:Minimum")) -> (number=w1196:dbl)  [unwired: 3 out]
                        n390 = property class="Slide (strict)"(reference=w1195, error in=w1194, "Scale.Range:Minimum"=w1196) -> (error out=w1198:errorcluster)  [unwired: 1 out]
                      }
                      frame "Maximum" {
                        n391 = Fract/Exp String To Number(string=w1201, default (0 dbl)=0.0 ("Data Range:Minimum")) -> (number=w1202:dbl)  [unwired: 3 out]
                        n392 = property class="Slide (strict)"(reference=w1200, error in=w1199, "Data Range:Maximum"=w1202) -> (error out=w1204:errorcluster)  [unwired: 1 out]
                      }
                      frame "Scale.Maximum" {
                        n393 = Fract/Exp String To Number(string=w1205, default (0 dbl)=0.0 ("Data Range:Minimum")) -> (number=w1208:dbl)  [unwired: 3 out]
                        n394 = property class="Slide (strict)"(reference=w1206, error in=w1207, "Scale.Range:Maximum"=w1208) -> (error out=w1210:errorcluster)  [unwired: 1 out]
                      }
                      frame "Increment" {
                        n395 = Fract/Exp String To Number(string=w1211, default (0 dbl)=0.0 ("Data Range:Minimum")) -> (number=w1214:dbl)  [unwired: 3 out]
                        n396 = property class="Slide (strict)"(reference=w1212, error in=w1213, "Data Range:Increment"=w1214) -> (error out=w1216:errorcluster)  [unwired: 1 out]
                      }
                      frame "Scale.Increment" {
                        n397 = Fract/Exp String To Number(string=w1217, default (0 dbl)=0.0 ("Data Range:Minimum")) -> (number=w1220:dbl)  [unwired: 3 out]
                        n398 = property class="Slide (strict)"(reference=w1218, error in=w1219, "Scale.Range:Increment"=w1220) -> (error out=w1222:errorcluster)  [unwired: 1 out]
                      }
                      frame "Scale.Start" {
                        n399 = Fract/Exp String To Number(string=w1224, default (0 dbl)=0.0 ("Data Range:Minimum")) -> (number=w1226:dbl)  [unwired: 3 out]
                        n400 = property class="Slide (strict)"(reference=w1223, error in=w1225, "Scale.Range:Start"=w1226) -> (error out=w1228:errorcluster)  [unwired: 1 out]
                      }
                      frame "Scale.MinorInc" {
                        n401 = Fract/Exp String To Number(string=w1229, default (0 dbl)=0.0 ("Data Range:Minimum")) -> (number=w1232:dbl)  [unwired: 3 out]
                        n402 = property class="Slide (strict)"(reference=w1231, error in=w1230, "Scale.Range:Minor Increment"=w1232) -> (error out=w1234:errorcluster)  [unwired: 1 out]
                      }
                      frame "Scale.Format String" {
                        n403 = property class="Slide (strict)"(reference=w1236, error in=w1237, "Scale.Format String"=w1235) -> (error out=w1238:errorcluster)  [unwired: 1 out]
                      }
                      frame "Scale.Format" {
                        n404 = Decimal String To Number(string=w1240, default (0L)=u8 0 ("Format & Precision:Format")) -> (number=w1242:u8)  [unwired: 2 out]
                        n405 = property class="Slide (strict)"(reference=w1239, error in=w1241, "Scale.Format & Precision:Format"=w1242) -> (error out=w1244:errorcluster)  [unwired: 1 out]
                      }
                      frame "Scale.Precision" {
                        n406 = Decimal String To Number(string=w1246, default (0L)=u8 0 ("Format & Precision:Format")) -> (number=w1248:u8)  [unwired: 2 out]
                        n407 = property class="Slide (strict)"(reference=w1247, error in=w1245, "Scale.Format & Precision:Precision"=w1248) -> (error out=w1250:errorcluster)  [unwired: 1 out]
                      }
                    }
                  }
                  frame 7 {
                    n408 = Type Cast(type=refnum<vi> refnum ("Slide"), x=w1257) -> (*(type *) &x=w1254:refnum<vi>)
                    n409 = case shown="\"Value\"" w1255 {
                      tunnel: [w1258 w1264 w1270 w1276 w1282 w1288 w1294 w1300 w1306 w1312 w1316 w1322 w1328] -> w1251
                      tunnel: w1254 -> [_ w1259 w1265 w1273 w1278 w1284 w1290 w1296 w1301 w1309 w1314 w1317 w1325]
                      tunnel: w1253 -> [w1258 w1261 w1267 w1272 w1277 w1285 w1291 w1297 w1303 w1308 w1315 w1319 w1323]
                      tunnel: w1252 -> [_ w1260 w1266 w1271 w1279 w1283 w1289 w1295 w1302 w1307 w1313 w1318 w1324]
                      frame "False", Default {
                      }
                      frame "Value" {
                        n410 = Fract/Exp String To Number(string=w1260, default (0 dbl)=u32 0) -> (number=w1263:u32)  [unwired: 3 out]
                        n411 = property class="Slide (strict)"(reference=w1259, error in=w1261, "Value"=w1263) -> (error out=w1264:errorcluster)  [unwired: 1 out]
                      }
                      frame "Minimum" {
                        n412 = Fract/Exp String To Number(string=w1266, default (0 dbl)=0.0 ("Data Range:Minimum")) -> (number=w1268:dbl)  [unwired: 3 out]
                        n413 = property class="Slide (strict)"(reference=w1265, error in=w1267, "Data Range:Minimum"=w1268) -> (error out=w1270:errorcluster)  [unwired: 1 out]
                      }
                      frame "Scale.Minimum" {
                        n414 = Fract/Exp String To Number(string=w1271, default (0 dbl)=0.0 ("Data Range:Minimum")) -> (number=w1274:dbl)  [unwired: 3 out]
                        n415 = property class="Slide (strict)"(reference=w1273, error in=w1272, "Scale.Range:Minimum"=w1274) -> (error out=w1276:errorcluster)  [unwired: 1 out]
                      }
                      frame "Maximum" {
                        n416 = Fract/Exp String To Number(string=w1279, default (0 dbl)=0.0 ("Data Range:Minimum")) -> (number=w1280:dbl)  [unwired: 3 out]
                        n417 = property class="Slide (strict)"(reference=w1278, error in=w1277, "Data Range:Maximum"=w1280) -> (error out=w1282:errorcluster)  [unwired: 1 out]
                      }
                      frame "Scale.Maximum" {
                        n418 = Fract/Exp String To Number(string=w1283, default (0 dbl)=0.0 ("Data Range:Minimum")) -> (number=w1286:dbl)  [unwired: 3 out]
                        n419 = property class="Slide (strict)"(reference=w1284, error in=w1285, "Scale.Range:Maximum"=w1286) -> (error out=w1288:errorcluster)  [unwired: 1 out]
                      }
                      frame "Increment" {
                        n420 = Fract/Exp String To Number(string=w1289, default (0 dbl)=0.0 ("Data Range:Minimum")) -> (number=w1292:dbl)  [unwired: 3 out]
                        n421 = property class="Slide (strict)"(reference=w1290, error in=w1291, "Data Range:Increment"=w1292) -> (error out=w1294:errorcluster)  [unwired: 1 out]
                      }
                      frame "Scale.Increment" {
                        n422 = Fract/Exp String To Number(string=w1295, default (0 dbl)=0.0 ("Data Range:Minimum")) -> (number=w1298:dbl)  [unwired: 3 out]
                        n423 = property class="Slide (strict)"(reference=w1296, error in=w1297, "Scale.Range:Increment"=w1298) -> (error out=w1300:errorcluster)  [unwired: 1 out]
                      }
                      frame "Scale.Start" {
                        n424 = Fract/Exp String To Number(string=w1302, default (0 dbl)=0.0 ("Data Range:Minimum")) -> (number=w1304:dbl)  [unwired: 3 out]
                        n425 = property class="Slide (strict)"(reference=w1301, error in=w1303, "Scale.Range:Start"=w1304) -> (error out=w1306:errorcluster)  [unwired: 1 out]
                      }
                      frame "Scale.MinorInc" {
                        n426 = Fract/Exp String To Number(string=w1307, default (0 dbl)=0.0 ("Data Range:Minimum")) -> (number=w1310:dbl)  [unwired: 3 out]
                        n427 = property class="Slide (strict)"(reference=w1309, error in=w1308, "Scale.Range:Minor Increment"=w1310) -> (error out=w1312:errorcluster)  [unwired: 1 out]
                      }
                      frame "Scale.Format String" {
                        n428 = property class="Slide (strict)"(reference=w1314, error in=w1315, "Scale.Format String"=w1313) -> (error out=w1316:errorcluster)  [unwired: 1 out]
                      }
                      frame "Scale.Format" {
                        n429 = Decimal String To Number(string=w1318, default (0L)=u8 0 ("Format & Precision:Format")) -> (number=w1320:u8)  [unwired: 2 out]
                        n430 = property class="Slide (strict)"(reference=w1317, error in=w1319, "Scale.Format & Precision:Format"=w1320) -> (error out=w1322:errorcluster)  [unwired: 1 out]
                      }
                      frame "Scale.Precision" {
                        n431 = Decimal String To Number(string=w1324, default (0L)=u8 0 ("Format & Precision:Format")) -> (number=w1326:u8)  [unwired: 2 out]
                        n432 = property class="Slide (strict)"(reference=w1325, error in=w1323, "Scale.Format & Precision:Precision"=w1326) -> (error out=w1328:errorcluster)  [unwired: 1 out]
                      }
                    }
                  }
                }
              }
              frame "Boolean" {
                n433 = Type Cast(type=refnum<vi> refnum ("Boolean 2"), x=w1333) -> (*(type *) &x=w1332:refnum<vi>)
                n434 = case shown="\"Value\"" w1329 {
                  tunnel: w1335 -> [w1336 w1342 w1346]
                  tunnel: [w1336 w1341 w1345] -> w1334
                  tunnel: w1332 -> [_ w1340 w1344]
                  tunnel: w1331 -> [_ w1338 w1343]
                  frame "False", Default {
                  }
                  frame "Value" {
                    n435 = Equal?(x=w1338, y="TRUE" ("x")) -> (x = y?=w1339:bool)
                    n436 = property class="Bool (strict)"(reference=w1340, error in=w1342, "Value"=w1339) -> (error out=w1341:errorcluster)  [unwired: 1 out]
                  }
                  frame "BooleanText" {
                    n437 = property class="Bool (strict)"(reference=w1344, error in=w1346, "Boolean Text.Text"=w1343) -> (error out=w1345:errorcluster)  [unwired: 1 out]
                  }
                }
              }
            }
          }
          frame -1 {
          }
        }
      }
      n438 = call "VI Server_Defer FP Update.vi"("Defer Panel Updates? (F)"=FALSE ("Defer Panel Updates (F)"), "error in"=w15, "VI Server Cluster"=w10) -> ("error out"=w16:errorcluster, "VI Server Cluster.DUP"=w12:T2)  [unwired: 7 out]
    }
    frame Error {
      n439 = call "VI Server_Empty VI Server Cluster.vi"() -> ("VI Server Cluster"=w1358:T2)  [unwired: 7 in]
    }
  }
  "error out" <- w7
  "VI Server Cluster.DUP" <- w3
  n440 = local write "VI Server.RefsCluster"(w1) -> ()
  n441 = Request Deallocation(w2) -> ()
